vi "Remove Quotes from String.vi"(11 "String in":string) -> (3 "String out":string)   [LabVIEW 2013, in "OPC UA Client System Explorer.lvlib"]
uses:
  OPC UA Client System Explorer.lvlib
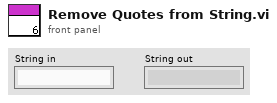
[diagram p1: front panel]
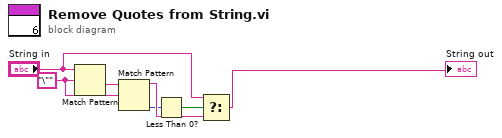
[diagram p0: block diagram]
diagram:
  w2 = "\"" ("regular expression")
  n1 = Match Pattern(string="String in", regular expression=w2) -> (after substring=w1:string)  [unwired: 1 in, 3 out]
  n2 = Match Pattern(string=w1, regular expression=w2) -> (before substring=w5:string, offset past match=w3:i32)  [unwired: 1 in, 2 out]
  n3 = Less Than 0?(x=w3) -> (x < 0?=w4:bool)
  n4 = Select(t="String in", s=w4, f=w5) -> (s? t:f=→"String out":string)
